vi "STM Command Based Example - Client.vi"() -> ()   [LabVIEW 2010]
doc: "This example demonstrates how to use STM with TCP to implement a command based communications application. \n\nThe client sends messages to the server on the type of signals to generate (frequency, FFT window type) and then receives time domain and spectral data from the server.\n\nThe server must be started first."
uses:
  vi.lib/NI/STM/TCP/TCP Read Options.ctl
  vi.lib/NI/STM/TCP/Read Meta Data (TCP Ref).vi
  vi.lib/NI/STM/TCP/Get Connection Reference (TCP).vi
  vi.lib/NI/STM/TCP/Write Message (TCP).vi
  vi.lib/NI/STM/TCP/Read Meta Data (TCP Clst).vi
  vi.lib/NI/STM/TCP/Read Message (TCP).vi
  vi.lib/NI/STM/NI STM.lvlib
panel:
  in  "Power Spectrum Window":T1(ring)=enum."Blackman-Harris"
  out "Processed  Data":cluster{"f0":dbl, "df":dbl, "magnitude":dbl[]}(graph)
  in  "Frequency":dbl(knob)=2000.0 scale=10.0..10000.0
  out "Acquired Data":waveform(dbl)(graph)
  in  "Target IP Address":string="localhost"
  in  "stop":bool
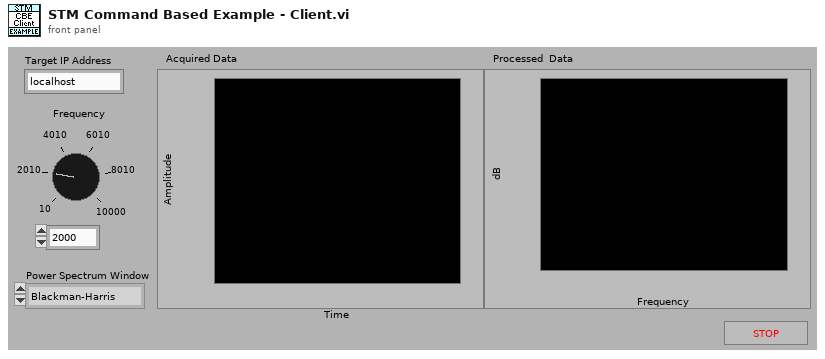
[diagram p1: front panel]
types:
  T1 = enum16{"None ", "Hanning", "Hamming", "Blackman-Harris", "Exact Blackman", "Blackman", "Flat Top", "4 Term B-Harris ", "7 Term B-Harris", "Low Sidelobe"}
  T2 = typedef "NI STM.lvlib/TCP Connection Info.ctl" = cluster{"connection ID":refnum<k5>, "meta data":T3[]}
  T3 = typedef "NI STM.lvlib/MetaDataElement.ctl" = string
  T4 = typedef "NI STM.lvlib/TCP Read Options.ctl" = cluster{"ignore timeout error":bool, "timeout ms (1000)":i32}
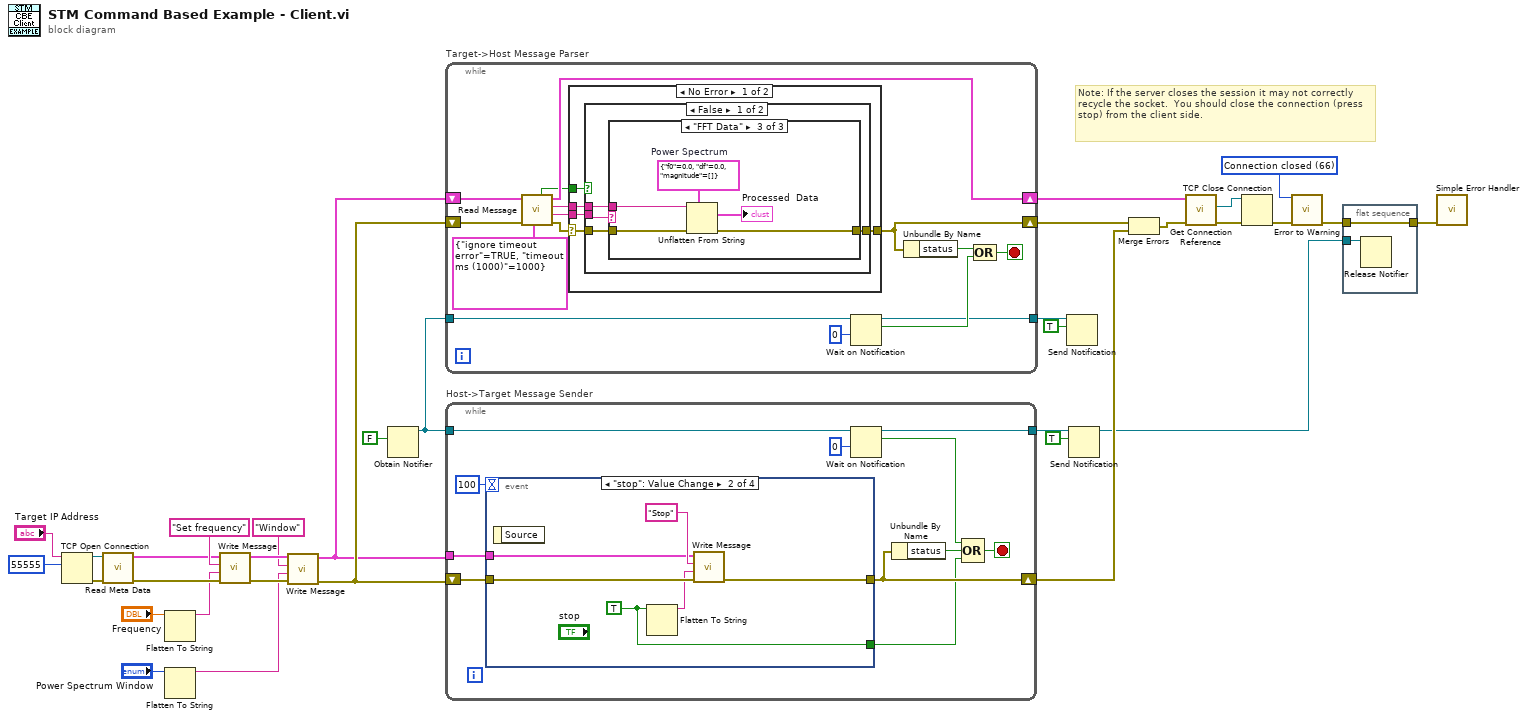
[diagram p0: block diagram]
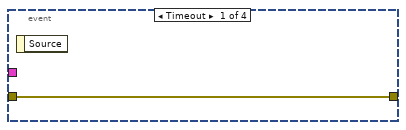
[diagram p2: hidden frame]
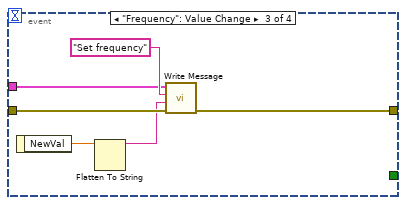
[diagram p3: hidden frame]
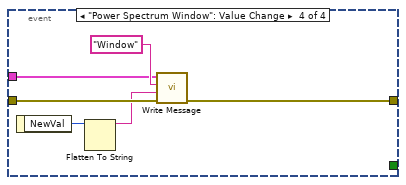
[diagram p4: hidden frame]
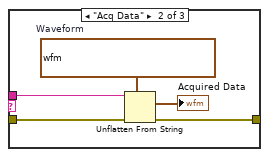
[diagram p6: hidden frame]
diagram:
  w29 = 66 items=["No Error", "Argument Error", "Memory Full", "Out of Zone", "End of File", "File Already Open", "Generic File IO Error", "File Not Found", "File Permission Error", "Disk Full", "Duplicate Path", "Too Many Files Open", "Not Enabled", "Resource File Not Found", "Cannot Add Resource", "Resource Not Found", "Image Not Found", "Image Memory Error", "Pen Does Not Exist", "Config Bad Type", "Config Token Not Found", "Config Parse Error", "Config Memory Error", "Bad External Code Format", "Bad External Code Offset", "External Code Not Present", "Null Window", "Destroy Window Mixup", "Null Menu", "Print Aborted", "Bad Print Record", "Print Driver Error", "Windows Error During Print", "Memory Error During Print", "Print Dialog Error", "Generic Print Error", "Invalid Device Refnum", "Device Not Found", "Device Parameter Error", "Device Unit Error", "Can't Open Device", "Device Call Aborted", "Generic Error", "Cancelled By User", "Object ID Too Low", "Object ID Too High", "Object Not In Heap", "Unknown Heap", "Bad DefProc ID", "DefProc Not In Table", "Message Out Of Range", "Null Method", "Unknown Message", "Manager Call Not Supported", "Bad address", "Connection In progress", "Connection timed out", "Connection is already in progress", "Network attribute not supported", "Network error", "Address in use", "System out of memory", "Connection aborted", "Connection refused", "Connection is not connected", "Connection is already connected", "Connection closed", "Initialize error (interapplication manager)", "Bad occurrence", "Wait on unbound occurrence handler", "Occurrence queue overflow", "Bad path", "Semaphore not signaled", "Unrecognized type (interapplication manager)"] ("1st Error to Convert")
  # "Note: If the server closes the session it may not correctly recycle the socket.  You should close the connection (press stop) from the client side."
  n1 = TCP Open Connection(address="Target IP Address", remote port or service name=u16 55555 ("remote port")) -> (connection ID=w33:refnum<k5>, error out=w32:errorcluster)  [unwired: 1 in, 2 out]
  n2 = call-poly "Read Meta Data.vi"("error in"=w32, "connection ID"=w33) -> ("error out"=w28:errorcluster, "connection info out"=w11:T2)  [unwired: 1 in, 7 out]
  n3 = Flatten To String(anything="Frequency") -> (data string=w20:string)  [unwired: 1 in, 4 out]
  n4 = Flatten To String(anything="Power Spectrum Window") -> (data string=w21:string)  [unwired: 2 in, 3 out]
  n5 = call-poly "Write Message.vi"("error in"=w28, "data"=w20, "name"="Set frequency" ("Name"), "connection info in"=w11) -> ("error out"=w25:errorcluster, "connection info out"=w26:T2)  [unwired: 1 in, 5 out]
  n6 = call-poly "Write Message.vi"("error in"=w25, "data"=w21, "name"="Window" ("Name"), "connection info in"=w26) -> ("error out"=w23:errorcluster, "connection info out"=w10:T2)  [unwired: 1 in, 5 out]
  n7 = Obtain Notifier(notification data type=FALSE) -> (notifier out=w8:refnum<notifier>)  [unwired: 3 in, 2 out]
  n8 = while "Target->Host Message Parser" {
    shift-right: [w46] -> w18
    shift-left: w10 -> [w48]
    shift-right: [w34] -> w14
    shift-left: w23 -> [w47]
    tunnel: w8 -> [w39]
    tunnel: [w37] -> w6
    stop <- w36 stop-if-true
    n9 = call-poly "Read Message.vi"("options"=T4 {"ignore timeout error"=TRUE, "timeout ms (1000)"=1000} ("Options"), "error in"=w47, "connection info in"=w48) -> ("error out"=w42:errorcluster, "name"=w45:T3, "data string"=w44:string, "connection info out"=w46:T2, "timed out?"=w43:bool)  [unwired: 2 in, 2 out]
    n10 = case shown="No Error" w42 {
      selector: w42 -> [w50 w70]
      tunnel: w45 -> [w53 _]
      tunnel: w44 -> [w52 _]
      tunnel: w43 -> [w51 _]
      tunnel: [w49 w70] -> w34
      frame No Error {
        n11 = case shown="False" w51 {
          tunnel: w53 -> [w54 _]
          tunnel: w52 -> [w57 _]
          tunnel: w50 -> [w56 w69]
          tunnel: [w55 w69] -> w49
          frame False {
            n12 = case shown="\"FFT Data\"" w54 {
              tunnel: w57 -> [_ w63 w68]
              tunnel: w56 -> [w58 w60 w65]
              tunnel: [w58 w59 w64] -> w55
              frame Default {
              }
              frame "Acq Data" {
                w62 = waveform(dbl) {"t0"=timestamp(0 s since 1904-01-01), "dt"=0.0, "Y"=[]}  # Waveform
                n13 = Unflatten From String(type=w62, binary string=w63, error in (no error)=w60) -> (value=→"Acquired Data":waveform(dbl), error out=w59:errorcluster)  [unwired: 3 out]
              }
              frame "FFT Data" {
                w67 = cluster{"f0":dbl, "df":dbl, "magnitude":dbl[]} {"f0"=0.0, "df"=0.0, "magnitude"=[]}  # Power Spectrum
                n14 = Unflatten From String(type=w67, binary string=w68, error in (no error)=w65) -> (value=→"Processed  Data":cluster{"f0":dbl, "df":dbl, "magnitude":dbl[]}, error out=w64:errorcluster)  [unwired: 3 out]
              }
            }
          }
          frame True {
          }
        }
      }
      frame Error {
      }
    }
    n15 = Wait on Notification(notifier=w39, timeout in ms (-1)=0) -> (notifier out=w37:refnum<notifier>, notification=w38:bool)  [unwired: 2 in, 2 out]
    n16 = Unbundle By Name(w34) -> ("status"=w35:bool)
    n17 = Compound Arithmetic op=OR(w35, w38) -> (w36:bool)
  }
  n18 = while "Host->Target Message Sender" {
    tunnel: w10 -> [w81]
    shift-right: [w76] -> w15
    shift-left: w23 -> [w80]
    tunnel: w8 -> [w77]
    tunnel: [w71] -> w4
    stop <- w73 stop-if-true
    n19 = event shown="[1] \"stop\": Value Change" {
      selector: _ -> [_ _ _ _]
      dyn-events: _ -> [_ _ _ _]
      timeout: 100 -> [_ _ _ _]
      tunnel: w81 -> [_ w87 w93 w98]
      tunnel: w80 -> [w82 w86 w92 w99]
      tunnel: [_ w84 _ _] -> w74
      tunnel: [w82 w83 w89 w95] -> w76
      event Timeout {
        n20 = event-data() -> ()  [unwired: 2 out]
      }
      event "stop": Value Change {
        w84 = TRUE ("stop")
        n21 = event-data() -> ()  [unwired: 2 out]
        n22 = Flatten To String(anything=w84) -> (data string=w85:string)  [unwired: 2 in, 3 out]
        n23 = call-poly "Write Message.vi"("error in"=w86, "data"=w85, "name"="Stop" ("Name"), "connection info in"=w87) -> ("error out"=w83:errorcluster)  [unwired: 1 in, 6 out]
      }
      event "Frequency": Value Change {
        n24 = event-data() -> ("NewVal"=w91:dbl)  [unwired: 1 out]
        n25 = Flatten To String(anything=w91) -> (data string=w90:string)  [unwired: 1 in, 4 out]
        n26 = call-poly "Write Message.vi"("error in"=w92, "data"=w90, "name"="Set frequency" ("Name"), "connection info in"=w93) -> ("error out"=w89:errorcluster)  [unwired: 1 in, 6 out]
      }
      event "Power Spectrum Window": Value Change {
        n27 = event-data() -> ("NewVal"=w97:T1)  [unwired: 1 out]
        n28 = Flatten To String(anything=w97) -> (data string=w96:string)  [unwired: 2 in, 3 out]
        n29 = call-poly "Write Message.vi"("error in"=w99, "data"=w96, "name"="Window" ("Name"), "connection info in"=w98) -> ("error out"=w95:errorcluster)  [unwired: 1 in, 6 out]
      }
    }
    n30 = Wait on Notification(notifier=w77, timeout in ms (-1)=0) -> (notifier out=w71:refnum<notifier>, notification=w72:bool)  [unwired: 2 in, 2 out]
    n31 = Unbundle By Name(w76) -> ("status"=w75:bool)
    n32 = Compound Arithmetic op=OR(w72, w75, w74) -> (w73:bool)
  }
  n33 = Send Notification(notification=TRUE, notifier=w6) -> ()  [unwired: 1 in, 2 out]
  n34 = Send Notification(notification=TRUE, notifier=w4) -> (notifier out=w1:refnum<notifier>)  [unwired: 1 in, 1 out]
  n35 = Merge Errors(w14, w15) -> (w13:errorcluster)
  n36 = call-poly "Get Connection Reference.vi"("error in"=w13, "connection info in"=w18) -> ("error out"=w16:errorcluster, "connection ID out"=w17:refnum<k5>)  [unwired: 8 out]
  n37 = TCP Close Connection(connection ID=w17, error in (no error)=w16) -> (error out=w12:errorcluster)  [unwired: 2 out]
  n38 = call <vilib>:"Error to Warning.vi"("1st Error to Convert"=w29, "error in"=w12) -> ("warning out"=w3:errorcluster)  [unwired: 3 in, 10 out]
  n39 = flat-sequence {
    tunnel: w1 -> [w102]
    tunnel: w3 -> [w101]
    tunnel: [w101] -> w2
    frame #0 {
      n40 = Release Notifier(notifier=w102) -> ()  [unwired: 2 in, 3 out]
    }
  }
  n41 = call <vilib>:"Simple Error Handler.vi"("error in (no error)"=w2) -> ()  [unwired: 4 in, 5 out]
